vi "OE1311&OE1351_Configure Channel Out.vi"(7 "OE1300_Configure Channel Out":T1={"CH2 Offset(%)"=0.0, "CH1 Offset(%)"=0.0, "CH2 Expand"=1, "CH1 Expand"=1, "AUX OUT1"=1.0, "AUX OUT2"=1.0, "CH 1"=3, "CH 2"=3} {"CH 2" items=["Fixed", "X", "Y", "R", "Theta", "Xh1", "Yh1", "Rh1", "Theta h1", "Xh2", "Yh2", "Rh2", "Theta h2", "Xh3", "Yh3", "Rh3", "Theta h3", "Rh4", "Xh4", "Yh4", "Theta h4", "Rh5", "Xh5", "Yh5", "Theta h5", "Rh6", "Xh6", "Yh6", "Theta h6", "Rh7", "Xh6", "Yh6", "Theta h7", "X_Noise", "Y_Noise", "Freq", "AuxIn1", "AuxIn2"]; "CH 1" items=["Fixed", "X", "Y", "R", "Theta", "Xh1", "Yh1", "Rh1", "Theta h1", "Xh2", "Yh2", "Rh2", "Theta h2", "Xh3", "Yh3", "Rh3", "Theta h3", "Rh4", "Xh4", "Yh4", "Theta h4", "Rh5", "Xh5", "Yh5", "Theta h5", "Rh6", "Xh6", "Yh6", "Theta h6", "Rh7", "Xh6", "Yh6", "Theta h7", "X_Noise", "Y_Noise", "Freq", "AuxIn1", "AuxIn2"]; "AUX OUT2" min=-10.0 max=10.0 format="%#.3g"; "AUX OUT1" min=-10.0 max=10.0 format="%#.3g"; "CH1 Expand" min=1 max=256; "CH2 Expand" min=1 max=256; "CH1 Offset(%)" min=-100.0 max=100.0 format="%#.2g"; "CH2 Offset(%)" min=-100.0 max=100.0 format="%#.2g"}, 8 "Error in (no error)":errorcluster caption="error out（no error）", 9 "Remote Mode":u16(ring)=1 items=["RS232"=1, "Ethernet"=3], 10 "Connection ID in":refnum<k5>, 11 "VISA resource name":refnum<visa-resource-name>) -> (0 "Error out":errorcluster caption="error out", 1 "Output String":string, 2 "Connection ID out":refnum<k5>, 3 "VISA resource  out":refnum<visa-resource-name>)   [LabVIEW 2011]
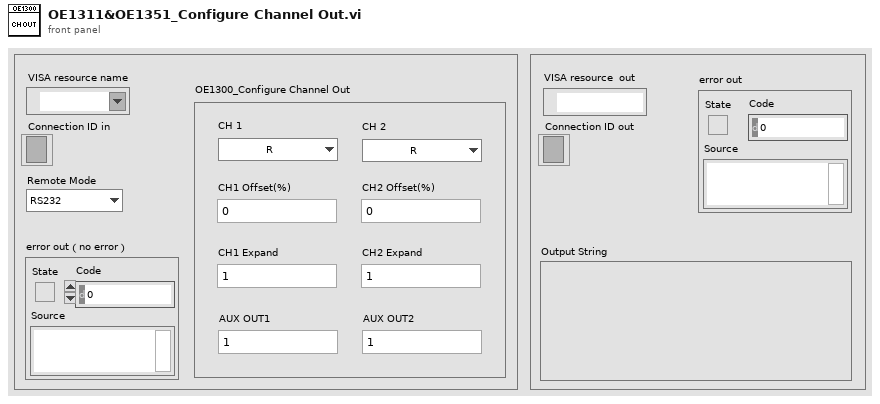
[diagram p1: front panel]
types:
  T1 = cluster{"CH2 Offset(%)":dbl, "CH1 Offset(%)":dbl, "CH2 Expand":i16, "CH1 Expand":i16, "AUX OUT1":dbl, "AUX OUT2":dbl, "CH 1":u16, "CH 2":u16}
  T2 = enum16{"ISRC", "IGND", "ICPL", "ILIN", "PHAS", "FMOD", "RSLP", "FREQ", "SWPT", "SLLM", "SULM", "SSLL", "SSLG", "STLM", "SWRM", "IRNG", "SENS", "RMOD", "OFLT", "OFSL", "SYNC", "DMOD", "HARM", "DARB", "SWVT", "SLVL", "SVLL", "SVUL", "SVSL", "SVSG", "SVTM", "SVRM", "RALL", "SNAP", "OUTP", "OAUX", "COUT", "CAUX", "COFP", "CEXP", "FPOP", "OEXP", "*IDN", "*RST", "OVLD", "INOV", "GNOV", "*PLL", "SSET", "RSET", "AGAN", "APHS", "ARSV", "ASCL", "EQCD", "EQCS", "SPED", "SRAT", "SLEN", "SSLE", "STRG", "SPRM", "STRD", "PAUS", "REST", "SPTS", "TRCA", "TEMP", "RSTU", "IHNZ", "DEQU", "SADD", "ARNG", "CSPE", "ISRCD", "IGNDD", "ICPLD", "ILIND", "PHASD", "FMODD", "RSLPD", "FREQD", "SWPTD", "SLLMD", "SULMD", "SSLLD", "SSLGD", "STLMD", "SWRMD", "SENSD", "RMODD", "OFLTD", "OFSLD", "SYNCD", "HARMD", "EQCDD", "EQCSD", "SNAPD", "OUTPD", "SWVTD", "SLVLD", "SVLLD", "SVULD", "SVSLD", "SVSGD", "SVTMD", "SVRMD", "SVDCD", "ARSVD", "AGAND", "APHSD", "ASCLD", "FPOPD", "CAUXD", "OEXPD", "SPEDD", "SRATD", "SLEND", "SSLED", "STRGD", "SPRMD", "STRDD", "PAUSD", "RESTD", "SPTSD", "TRCAD", "*IDND", "*RSTD", "INOVD", "GNOVD", "*PLLD", "SSETD", "RSETD", "RALLD"}
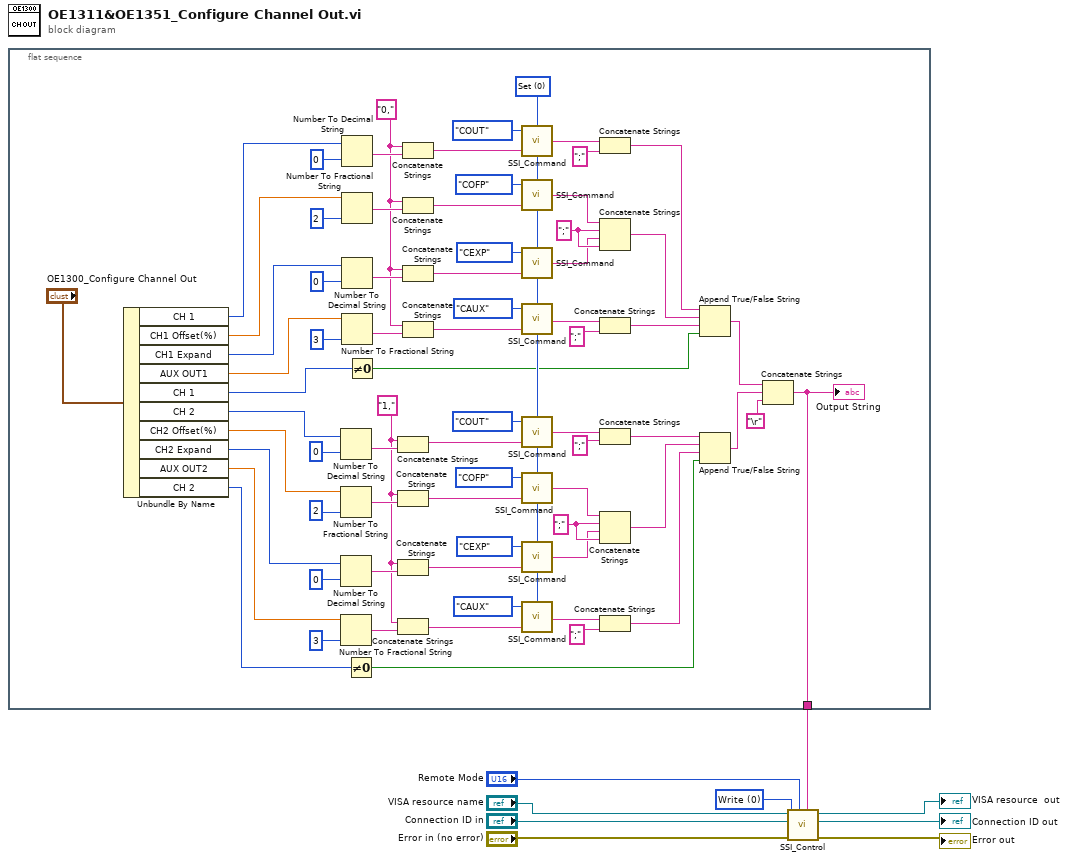
[diagram p0: block diagram]
diagram:
  w7 = u16 0 items=["Write", "Read"] ("Control")
  n1 = flat-sequence {
    tunnel: [w28] -> w1
    frame #0 {
      w10 = "1,"
      w19 = "0,"
      w58 = ";" ("替换字符串(\"\")")
      w72 = ";" ("替换字符串(\"\")")
      w40 = u16 0 items=["Set", "Query"] ("Opera")
      n2 = Unbundle By Name("OE1300_Configure Channel Out") -> ("CH 1"=w43:u16, "CH1 Offset(%)"=w42:dbl, "CH1 Expand"=w39:i16, "AUX OUT1"=w36:dbl, "CH 1"=w37:u16, "CH 2"=w35:u16, "CH2 Offset(%)"=w30:dbl, "CH2 Expand"=w31:i16, "AUX OUT2"=w32:dbl, "CH 2"=w33:u16)
      n3 = Number To Decimal String(number=w35, width (-)=i16 0 ("精度(6)")) -> (decimal integer string=w11:string)
      n4 = Number To Fractional String(number=w30, precision (6)=i16 2 ("精度(6)")) -> (F-format string=w12:string)  [unwired: 2 in]
      n5 = Number To Decimal String(number=w31, width (-)=i16 0 ("精度(6)")) -> (decimal integer string=w13:string)
      n6 = Number To Fractional String(number=w32, precision (6)=i16 3 ("精度(6)")) -> (F-format string=w14:string)  [unwired: 2 in]
      n7 = Number To Decimal String(number=w43, width (-)=i16 0 ("精度(6)")) -> (decimal integer string=w27:string)
      n8 = Number To Fractional String(number=w42, precision (6)=i16 2 ("精度(6)")) -> (F-format string=w25:string)  [unwired: 2 in]
      n9 = Number To Decimal String(number=w39, width (-)=i16 0 ("精度(6)")) -> (decimal integer string=w21:string)
      n10 = Number To Fractional String(number=w36, precision (6)=i16 3 ("精度(6)")) -> (F-format string=w20:string)  [unwired: 2 in]
      n11 = Not Equal To 0?(x=w33) -> (x != 0?=w34:bool)
      n12 = Not Equal To 0?(x=w37) -> (x != 0?=w38:bool)
      n13 = Concatenate Strings(w10, w11) -> (w18:string)
      n14 = Concatenate Strings(w10, w12) -> (w17:string)
      n15 = Concatenate Strings(w10, w13) -> (w16:string)
      n16 = Concatenate Strings(w10, w14) -> (w15:string)
      n17 = Concatenate Strings(w19, w27) -> (w26:string)
      n18 = Concatenate Strings(w19, w25) -> (w24:string)
      n19 = Concatenate Strings(w19, w21) -> (w23:string)
      n20 = Concatenate Strings(w19, w20) -> (w22:string)
      n21 = call "SSI_Command.vi"("Opera"=w40, "Paramter"=w26, "Command Type"=T2."COUT") -> ("Output string"=w69:string)  [unwired: 1 in]
      n22 = call "SSI_Command.vi"("Opera"=w40, "Paramter"=w24, "Command Type"=T2."COFP") -> ("Output string"=w79:string)  [unwired: 1 in]
      n23 = call "SSI_Command.vi"("Opera"=w40, "Paramter"=w23, "Command Type"=T2."CEXP") -> ("Output string"=w41:string)  [unwired: 1 in]
      n24 = call "SSI_Command.vi"("Opera"=w40, "Paramter"=w22, "Command Type"=T2."CAUX") -> ("Output string"=w75:string)  [unwired: 1 in]
      n25 = call "SSI_Command.vi"("Opera"=w40, "Paramter"=w18, "Command Type"=T2."COUT") -> ("Output string"=w55:string)  [unwired: 1 in]
      n26 = call "SSI_Command.vi"("Opera"=w40, "Paramter"=w17, "Command Type"=T2."COFP") -> ("Output string"=w64:string)  [unwired: 1 in]
      n27 = call "SSI_Command.vi"("Opera"=w40, "Paramter"=w16, "Command Type"=T2."CEXP") -> ("Output string"=w29:string)  [unwired: 1 in]
      n28 = call "SSI_Command.vi"("Opera"=w40, "Paramter"=w15, "Command Type"=T2."CAUX") -> ("Output string"=w61:string)  [unwired: 1 in]
      n29 = Concatenate Strings(w69, ";" ("替换字符串(\"\")")) -> (w68:string)
      n30 = Concatenate Strings(w79, w72, w41, w72) -> (w71:string)
      n31 = Concatenate Strings(w75, ";" ("替换字符串(\"\")")) -> (w73:string)
      n32 = Concatenate Strings(w55, ";" ("替换字符串(\"\")")) -> (w54:string)
      n33 = Concatenate Strings(w64, w58, w29, w58) -> (w57:string)
      n34 = Concatenate Strings(w61, ";" ("替换字符串(\"\")")) -> (w59:string)
      n35 = Append True/False String(1:w38, 2:w73, 3:w71, 4:w68) -> (0:w67:string)
      n36 = Append True/False String(1:w34, 2:w59, 3:w57, 4:w54) -> (0:w53:string)
      n37 = Concatenate Strings(w67, w53, "\r") -> (w28:string)
      "Output String" <- w28
    }
  }
  n38 = call "SSI_Control.vi"("Write Buffer"=w1, "Remote Mode"="Remote Mode", "Error in (no error)"="Error in (no error)", "Control"=w7, "Connection ID in"="Connection ID in", "VISA resource name"="VISA resource name") -> ("Error out"=→"Error out":errorcluster, "Connection ID out"=→"Connection ID out":refnum<k5>, "VISA resource  out"=→"VISA resource  out":refnum<visa-resource-name>)  [unwired: 2 in, 1 out]
